vi "Read Output.vi"(8 "error in (no error)":errorcluster, 11 "Fit Exponential in":refnum<class "Fit Exponential.lvclass">) -> (0 "error out":errorcluster, 2 "Output":T1, 3 "Fit Exponential out":refnum<class "Fit Exponential.lvclass">)   [LabVIEW 2012, in "Exponential Fit Library.lvlib" / "Fit Exponential.lvclass"]
uses:
  Fit Exponential.lvclass
  Fit Exponential.lvclass/Fit Exponential.ctl
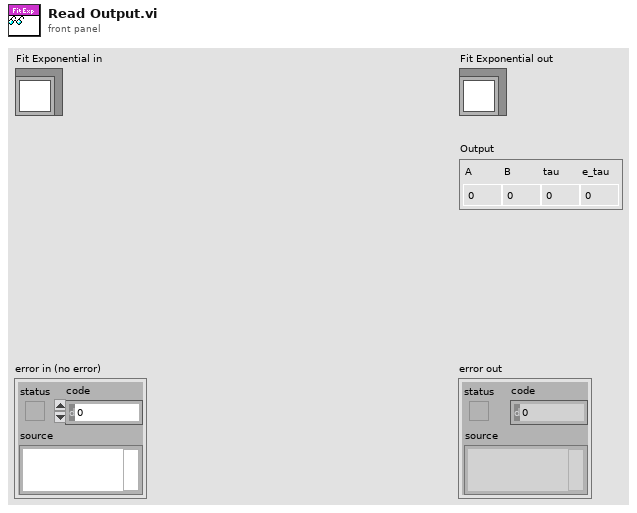
[diagram p1: front panel]
types:
  T1 = cluster{"A":dbl, "B":dbl, "tau":dbl, "e_tau":dbl}
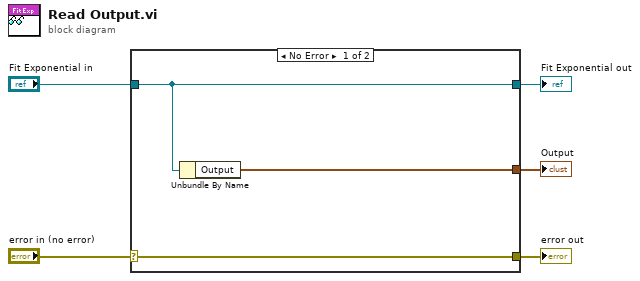
[diagram p0: block diagram]
diagram:
  n1 = case shown="No Error" "error in (no error)" {
    selector: "error in (no error)" -> [w8 w9]
    tunnel: [w8 w9] -> w4
    tunnel: [w7 w10] -> w2
    tunnel: "Fit Exponential in" -> [w7 w10]
    tunnel: [w6 _] -> w1
    frame No Error {
      n2 = Unbundle By Name(w7) -> ("Output"=w6:T1)
    }
    frame Error {
    }
  }
  "error out" <- w4
  "Fit Exponential out" <- w2
  "Output" <- w1
